vi "Init Configuration Parameters.vi"(8 "error in (no error)":errorcluster, 10 "Node Config":string, 11 "Node in":refnum<class "AMS Chiller Template.lvclass"> caption="Timed Node in") -> (0 "error out":errorcluster, 3 "Node out":refnum<class "AMS Chiller Template.lvclass"> caption="Timed Node out")   [LabVIEW 2026, in "AMS Chiller Template.lvlib" / "AMS Chiller Template.lvclass"]
uses:
  AMS Chiller Template.lvclass
  Configuration Params.ctl
  <vilib>/ADAS Replay HIL/Template Node/Plugin/Template Node/Common Configuration Params.ctl
  AMS Chiller Template.lvclass/AMS Chiller Template.ctl
  c3f9980b-0202-4a5c-a15f-679fa66f24a8.vi
  <vilib>/ADAS Replay HIL/AdasCommonUtilities/Config/Data Converter/SubVIs/Replace JSON SubArray with String.vi
  <vilib>/ADAS Replay HIL/AdasCommonUtilities/Config/Data Converter/SubVIs/Variant From Data Node.vi
  <vilib>/ADAS Replay HIL/Template Node/Plugin/Template Node/Write Common Config Params.vi
  <vilib>/ADAS Replay HIL/Template Node/Plugin/Template Node/Template Node.lvclass
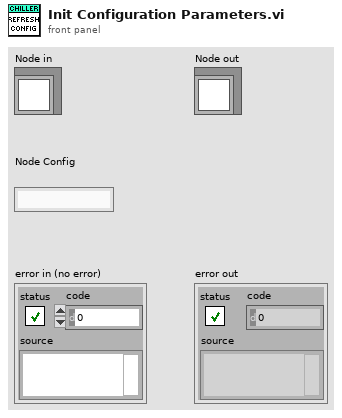
[diagram p1: front panel]
types:
  T1 = typedef "AMS Chiller Template.lvlib/AMS Chiller Template.lvclass/Configuration Params.ctl" = cluster{"Common":T2, "Amount of Channels":u32, "Address":string}
  T2 = typedef "Template Node.lvlib/Template Node.lvclass/Common Configuration Params.ctl" = cluster{"Iteration Interval (s)":dbl, "T0 (ns)":u64, "Priority":i32, "Processor":i32, "Wait in Ready State":bool}
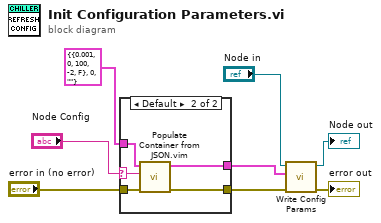
[diagram p0: block diagram]
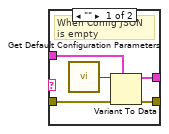
[diagram p2: hidden frame]
diagram:
  n1 = case shown="Default" "Node Config" {
    selector: "Node Config" -> [_ w14]
    tunnel: [w12 w18] -> w7
    tunnel: [w9 w17] -> w6
    tunnel: "error in (no error)" -> [w13 w16]
    tunnel: T1 {"Common"={"Iteration Interval (s)"=0.001, "T0 (ns)"=0, "Priority"=100, "Processor"=-2, "Wait in Ready State"=FALSE}, "Amount of Channels"=0, "Address"=""} ("Default Parameters") -> [w10 w15]
    frame "" {
      # "When Config JSON is empty"
      n2 = call "Get Default Configuration Parameters.vi"() -> ("Default Config Params"=w11:variant)
      n3 = Variant To Data(error in=w13, type=w10, Variant=w11) -> (data=w9:T1, error out=w12:errorcluster)
    }
    frame Default {
      n4 = call "Populate Container from JSON.vim"("error in (no error)"=w16, "JSON string In"=w14, "Container In"=w15) -> ("error out"=w18:errorcluster, "Container Out"=w17:T1)  [unwired: 6 in, 1 out]
    }
  }
  n5 = call "Write Config Params.vi"("error in"=w7, "Default Parameters"=w6, "Node in"="Node in") -> ("error out"=→"error out":errorcluster, "Node out"=→"Node out":refnum<class "AMS Chiller Template.lvclass">)  [unwired: 7 in]
